vi "GraphCom.vi"() -> ()   [LabVIEW 2019]
uses:
  MessageFormat1.ctl
  <vilib>/Instr/_visa.llb/VISA Configure Serial Port (Instr).vi
panel:
  in  "Tab Control":enum32{"Alcohol Test", "Configuration"}(tab)
  out "Horizontal Graduated Bar":u8(slide) scale=0.0..100.0
  out "RxData As Number":u32
  in  "Start Test":bool
  in  "stop":bool
  out "RxData Log":string
  in  "Disconnect from Arduino":bool
  in  "Connect to Arduino":bool
  in  "VISA resource name":refnum<visa-resource-name>
  out "Connected":bool
  out "Receiving Data":bool
  out "Input buffer":string
  in  "Stop Acquisition":bool
  # "Dades rebudes per UART"
  # "Dades transportades al Consumer Loop"
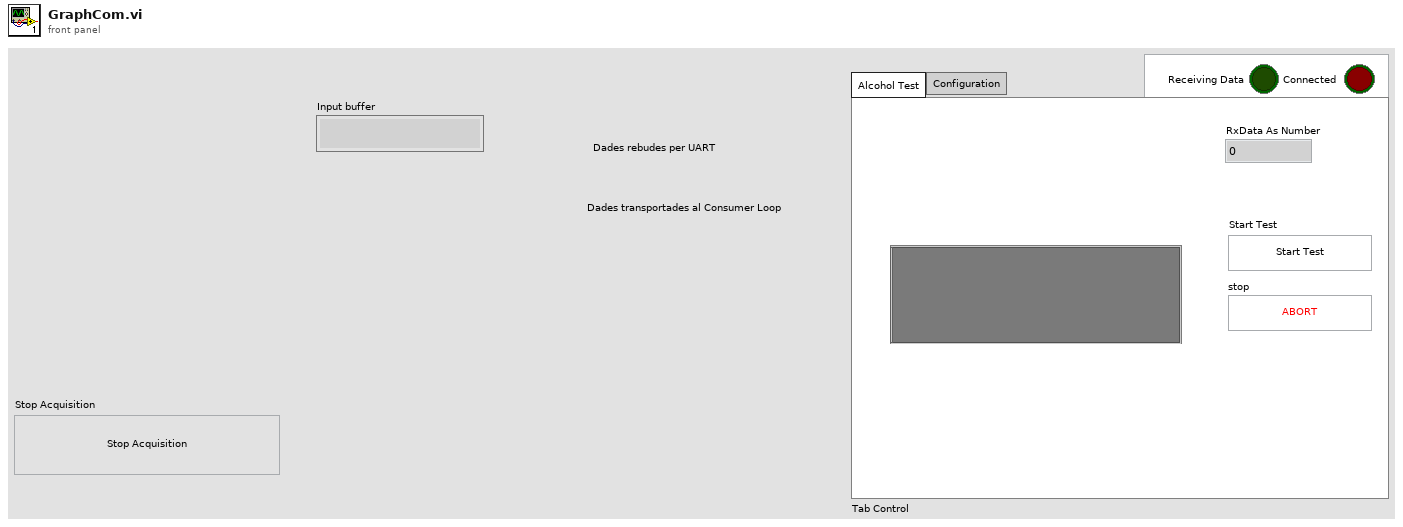
[diagram p1: front panel]
types:
  T1 = typedef "MessageFormat1.ctl" = cluster{"Consumer State":string, "RxData":string, "error constant":errorcluster, "Connected":bool, "Receiving Data":bool, "Producer State ":string}
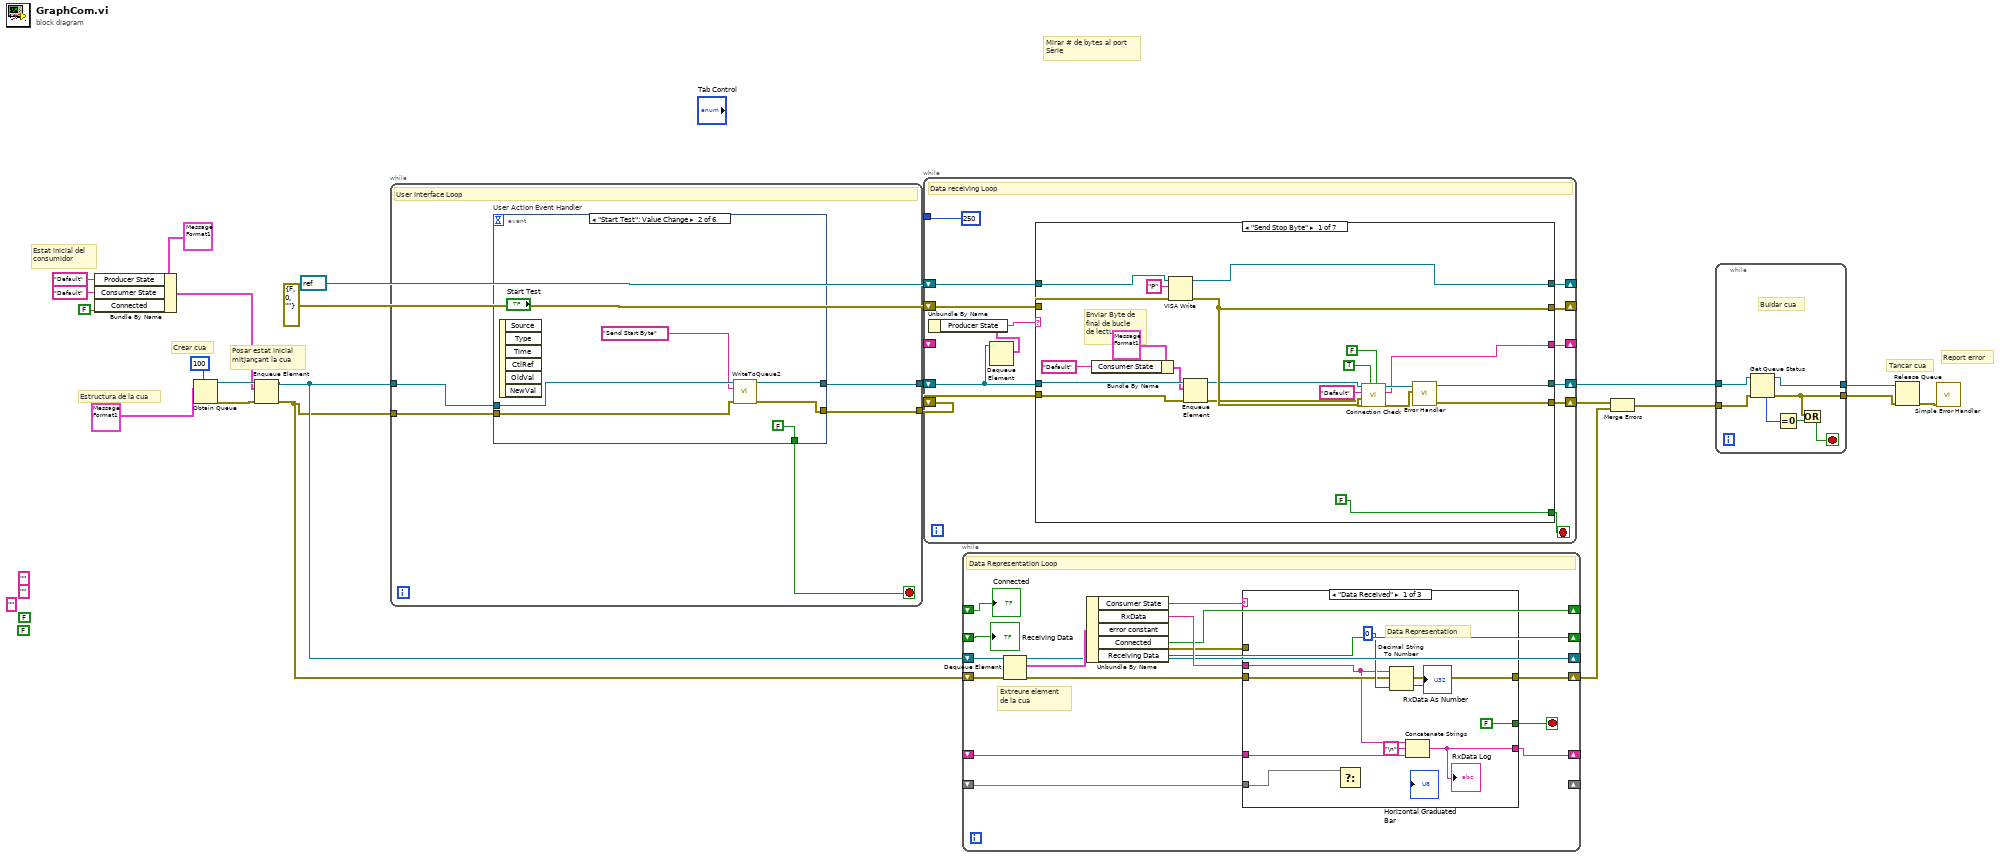
[diagram p0: block diagram]
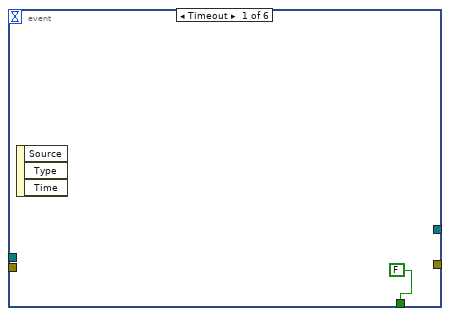
[diagram p2: hidden frame]
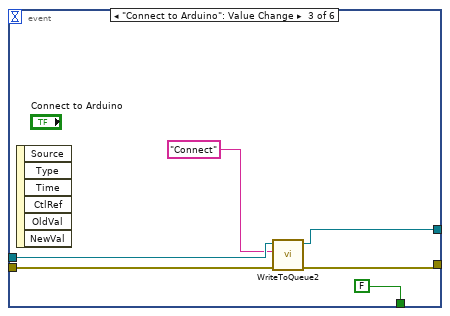
[diagram p3: hidden frame]
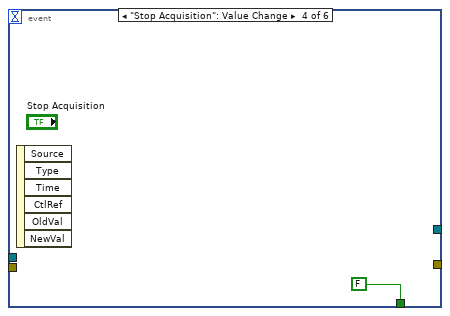
[diagram p4: hidden frame]
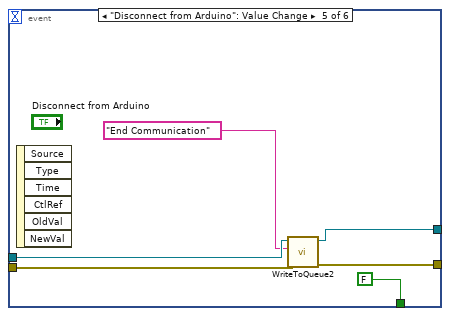
[diagram p5: hidden frame]
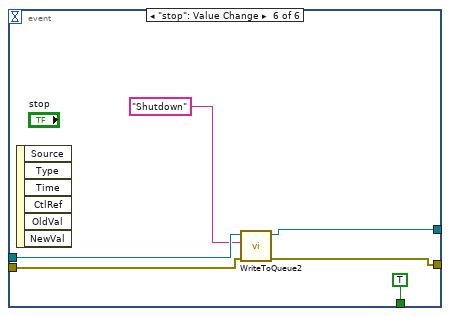
[diagram p6: hidden frame]
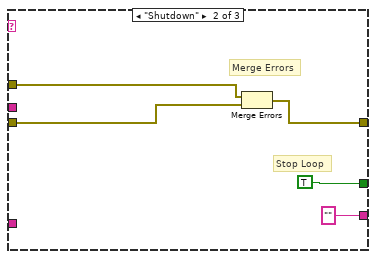
[diagram p7: hidden frame]
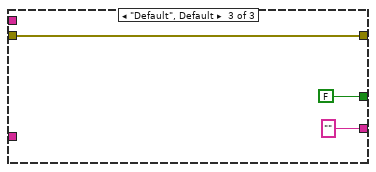
[diagram p8: hidden frame]
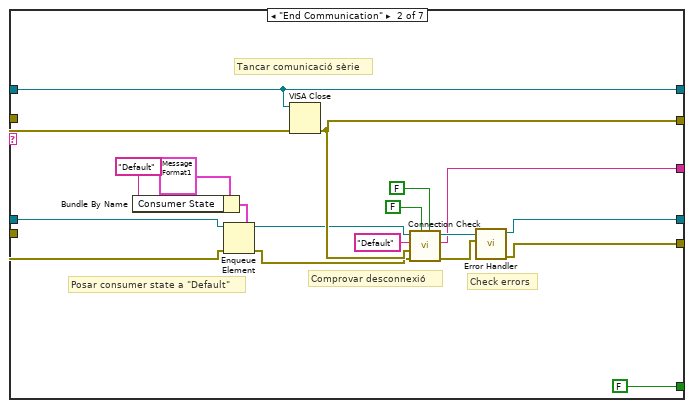
[diagram p9: hidden frame]
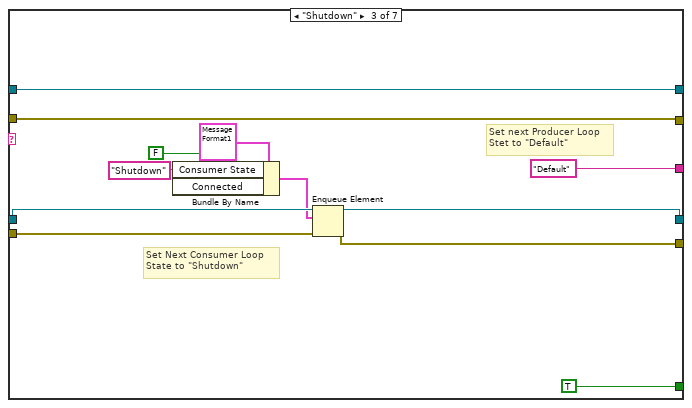
[diagram p10: hidden frame]
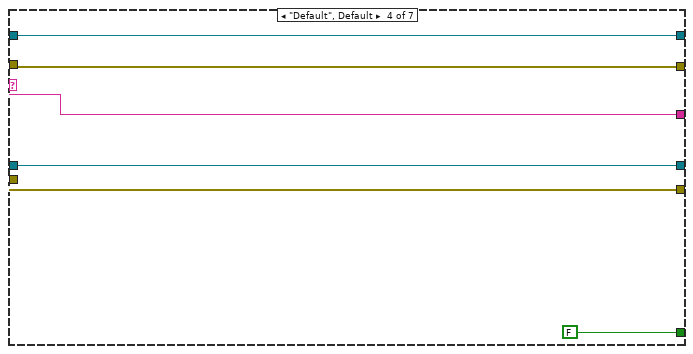
[diagram p11: hidden frame]
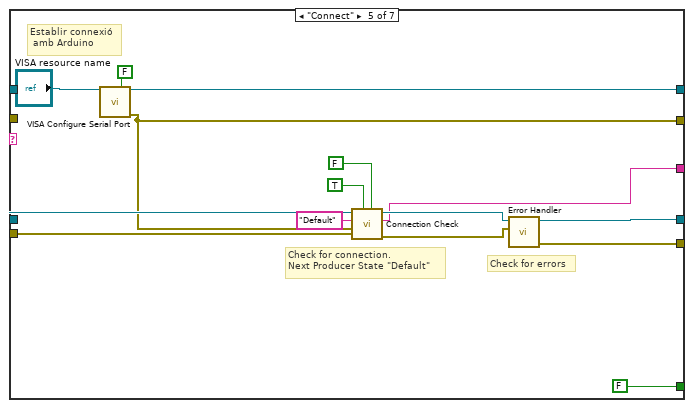
[diagram p12: hidden frame]
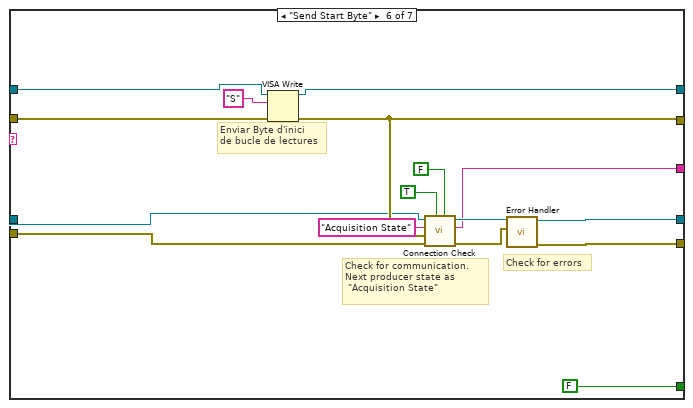
[diagram p13: hidden frame]
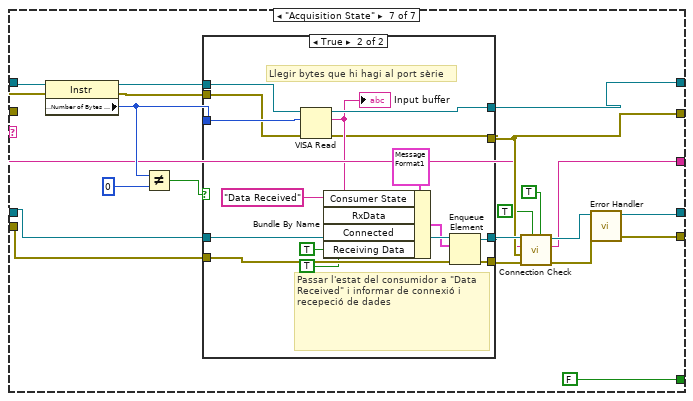
[diagram p14: hidden frame]
diagram:
  (unwired) "" ("Producer State")
  (unwired) FALSE ("Receiving Data")
  (unwired) FALSE ("Connected")
  (unwired) "" ("Consumer State")
  (unwired) "" ("Producer State")
  # "Tancar cua"
  # "Report error"
  # "Posar estat inicial \nmitjançant la cua"
  # "Crear cua"
  # "Mirar # de bytes al port\nSèrie"
  # "Estat inicial del \nconsumidor"
  # "Estructura de la cua"
  n1 = Bundle By Name(cluster=T1 {"Consumer State"="Consumer State", "RxData"="Received Data", "error constant"={"status"=FALSE, "code"=0, "source"=""}, "Connected"=FALSE, "Receiving Data"=FALSE, "Producer State "="Producer State"} ("Queue Definition"), "Producer State"="Default", "Consumer State"="Default", "Connected"=FALSE) -> (w15:T1)
  n2 = Obtain Queue(max queue size (-1, unlimited)=100, element data type=T1 {"Consumer State"="Consumer State", "RxData"="Received Data", "error constant"={"status"=FALSE, "code"=0, "source"=""}, "Connected"=FALSE, "Receiving Data"=FALSE, "Producer State "="Producer State"} ("Queue Definition")) -> (queue out=w17:refnum<queue>, error out=w18:errorcluster)  [unwired: 3 in, 1 out]
  n3 = Enqueue Element(queue=w17, element=w15, error in (no error)=w18) -> (queue out=w4:refnum<queue>, error out=w3:errorcluster)  [unwired: 1 in, 1 out]
  n4 = while {
    tunnel: w4 -> [w27]
    tunnel: w3 -> [w26]
    tunnel: [w25] -> w2
    tunnel: [w24] -> w1
    stop <- w23 stop-if-true
    # "User Interface Loop"
    n5 = event "User Action Event Handler" shown="[1] \"Start Test\": Value Change" {
      selector: _ -> [_ _ _ _ _ _]
      dyn-events: _ -> [_ _ _ _ _ _]
      timeout: _ -> [_ _ _ _ _ _]
      tunnel: w27 -> [_ w33 w40 _ w47 w52]
      tunnel: w26 -> [_ w34 w39 _ w46 w53]
      tunnel: [_ w32 w37 _ w44 w51] -> w25
      tunnel: [_ w31 w38 _ w43 w50] -> w24
      tunnel: [FALSE FALSE FALSE FALSE FALSE TRUE] -> w23
      event Timeout {
        n6 = event-data() -> ()  [unwired: 1 in, 3 out]
      }
      event "Start Test": Value Change {
        n7 = event-data() -> ()  [unwired: 1 in, 6 out]
        n8 = call "WriteToQueue2.vi"("error in (no error)"=w34, "Producer State"="Send Start Byte", "queue"=w33) -> ("error out"=w31:errorcluster, "queue out"=w32:refnum<queue>)  [unwired: 7 in]
      }
      event "Connect to Arduino": Value Change {
        n9 = event-data() -> ()  [unwired: 1 in, 6 out]
        n10 = call "WriteToQueue2.vi"("error in (no error)"=w39, "Producer State"="Connect" ("f"), "queue"=w40) -> ("error out"=w38:errorcluster, "queue out"=w37:refnum<queue>)  [unwired: 7 in]
      }
      event "Stop Acquisition": Value Change {
        n11 = event-data() -> ()  [unwired: 1 in, 6 out]
      }
      event "Disconnect from Arduino": Value Change {
        n12 = event-data() -> ()  [unwired: 1 in, 6 out]
        n13 = call "WriteToQueue2.vi"("error in (no error)"=w46, "Producer State"="End Communication" ("Producer State Out"), "queue"=w47) -> ("error out"=w43:errorcluster, "queue out"=w44:refnum<queue>)  [unwired: 7 in]
      }
      event "stop": Value Change {
        n14 = event-data() -> ()  [unwired: 1 in, 6 out]
        n15 = call "WriteToQueue2.vi"("error in (no error)"=w53, "Producer State"="Shutdown", "queue"=w52) -> ("error out"=w50:errorcluster, "queue out"=w51:refnum<queue>)  [unwired: 7 in]
      }
    }
  }
  n16 = while {
    shift-right: [w66] -> _
    shift-left: refnum<visa-resource-name> refnum ("VISA resource name out") -> [w63]
    shift-right: [w65] -> _
    shift-left: errorcluster {"status"=FALSE, "code"=0, "source"=""} ("error out") -> [w62]
    shift-right: [w58] -> w10
    shift-left: w2 -> [w56]
    shift-right: [w59] -> w21
    shift-left: w1 -> [w61]
    shift-right: [w64] -> _
    shift-left: _ -> [_]
    tunnel: [250] -> _
    stop <- w60 stop-if-true
    # "Data receiving Loop"
    n17 = Dequeue Element(queue=w56) -> (element=w55:T1)  [unwired: 2 in, 3 out]
    n18 = Unbundle By Name(w55) -> ("Producer State"=w54:string)
    n19 = case shown="\"Send Stop Byte\"" w54 {
      selector: w54 -> [_ _ _ w121 _ _ w159]
      tunnel: [w83 w104 w117 w122 w136 w152 w172] -> w66
      tunnel: [w74 w97 w116 w123 w130 w146 w162] -> w65
      tunnel: [w79 w96 w111 w124 w131 w150 w161] -> w59
      tunnel: [w80 w95 w112 w119 w132 w149 w160] -> w58
      tunnel: [FALSE FALSE TRUE FALSE FALSE FALSE FALSE] -> w60
      tunnel: [w78 w98 "Default" ("f") w121 w128 w145 w158] -> w64
      tunnel: w63 -> [w84 w104 w117 w122 _ w153 w177]
      tunnel: w62 -> [w85 w105 w116 w123 _ w154 w176]
      tunnel: w61 -> [w72 w92 w110 w124 w135 w143 w170]
      tunnel: w56 -> [w71 w93 w114 w119 w134 w142 w171]
      frame "Send Stop Byte" {
        # "Enviar Byte de \nfinal de bucle \nde lectures"
        n20 = Bundle By Name(cluster=T1 {"Consumer State"="Consumer State", "RxData"="Received Data", "error constant"={"status"=FALSE, "code"=0, "source"=""}, "Connected"=FALSE, "Receiving Data"=FALSE, "Producer State "="Consumer State"} ("Queue Definition"), "Consumer State"="Default") -> (w69:T1)
        n21 = VISA Write(VISA resource name=w84, write buffer="P", error in (no error)=w85) -> (VISA resource name out=w83:refnum<visa-resource-name>, error out=w74:errorcluster)  [unwired: 1 out]
        n22 = Enqueue Element(queue=w71, element=w69, error in (no error)=w72) -> (queue out=w70:refnum<queue>, error out=w73:errorcluster)  [unwired: 1 in, 1 out]
        n23 = call "Connection Check.vi"("Queue in"=w70, "Producer State In"="Default", "error in"=w74, "error in (no error)"=w73, "Connected"=TRUE, "Receiving Data"=FALSE) -> ("Queue out"=w82:refnum<queue>, "Producer State Out"=w78:string, "error out"=w81:errorcluster)  [unwired: 2 in]
        n24 = call "Error Handler.vi"("error in"=w81, "Queue in"=w82) -> ("error out"=w79:errorcluster, "Queue out"=w80:refnum<queue>)  [unwired: 8 in]
      }
      frame "End Communication" {
        # "Tancar comunicació sèrie"
        # "Check errors"
        # "Comprovar desconnexió"
        # "Posar consumer state a \"Default\""
        n25 = Bundle By Name(cluster=T1 {"Consumer State"="Consumer State", "RxData"="Received Data", "error constant"={"status"=FALSE, "code"=0, "source"=""}, "Connected"=FALSE, "Receiving Data"=FALSE, "Producer State "="Consumer State"} ("Queue Definition"), "Consumer State"="Default") -> (w88:T1)
        n26 = Enqueue Element(queue=w93, element=w88, error in (no error)=w92) -> (queue out=w94:refnum<queue>, error out=w91:errorcluster)  [unwired: 1 in, 1 out]
        n27 = VISA Close(VISA resource name=w104, error in (no error)=w105) -> (error out=w97:errorcluster)
        n28 = call "Connection Check.vi"("Queue in"=w94, "Producer State In"="Default", "error in"=w97, "error in (no error)"=w91, "Connected"=FALSE, "Receiving Data"=FALSE) -> ("Queue out"=w103:refnum<queue>, "Producer State Out"=w98:string, "error out"=w102:errorcluster)  [unwired: 2 in]
        n29 = call "Error Handler.vi"("error in"=w102, "Queue in"=w103) -> ("error out"=w96:errorcluster, "Queue out"=w95:refnum<queue>)  [unwired: 8 in]
      }
      frame "Shutdown" {
        # "Set next Producer Loop\nStet to \"Default\""
        # "Set Next Consumer Loop\nState to \"Shutdown\""
        n30 = Bundle By Name(cluster=T1 {"Consumer State"="Consumer State", "RxData"="Received Data", "error constant"={"status"=FALSE, "code"=0, "source"=""}, "Connected"=FALSE, "Receiving Data"=FALSE, "Producer State "="Consumer State"} ("Queue Definition"), "Consumer State"="Shutdown", "Connected"=FALSE) -> (w108:T1)
        n31 = Enqueue Element(queue=w114, element=w108, error in (no error)=w110) -> (queue out=w112:refnum<queue>, error out=w111:errorcluster)  [unwired: 1 in, 1 out]
      }
      frame "Default", Default {
      }
      frame "Connect" {
        # "Check for errors"
        # "Check for connection.\nNext Producer State \"Default\""
        # "Establir connexió\n amb Arduino"
        n32 = call-poly "VISA Configure Serial Port"("VISA resource name"="VISA resource name", "Enable Termination\nChar (T)"=FALSE ("Enable Termination\nChar (T)")) -> ("VISA resource name out"=w136:refnum<visa-resource-name>, "error out"=w130:errorcluster)  [unwired: 12 in]
        n33 = call "Connection Check.vi"("Queue in"=w134, "Producer State In"="Default", "error in"=w130, "error in (no error)"=w135, "Connected"=TRUE, "Receiving Data"=FALSE) -> ("Queue out"=w133:refnum<queue>, "Producer State Out"=w128:string, "error out"=w129:errorcluster)  [unwired: 2 in]
        n34 = call "Error Handler.vi"("error in"=w129, "Queue in"=w133) -> ("error out"=w131:errorcluster, "Queue out"=w132:refnum<queue>)  [unwired: 8 in]
      }
      frame "Send Start Byte" {
        # "Check for errors"
        # "Check for communication.\nNext producer state as\n \"Acquisition State\""
        # "Enviar Byte d'inici\nde bucle de lectures"
        n35 = VISA Write(VISA resource name=w153, write buffer="S", error in (no error)=w154) -> (VISA resource name out=w152:refnum<visa-resource-name>, error out=w146:errorcluster)  [unwired: 1 out]
        n36 = call "Connection Check.vi"("Queue in"=w142, "Producer State In"="Acquisition State", "error in"=w146, "error in (no error)"=w143, "Connected"=TRUE, "Receiving Data"=FALSE) -> ("Queue out"=w147:refnum<queue>, "Producer State Out"=w145:string, "error out"=w148:errorcluster)  [unwired: 2 in]
        n37 = call "Error Handler.vi"("error in"=w148, "Queue in"=w147) -> ("error out"=w150:errorcluster, "Queue out"=w149:refnum<queue>)  [unwired: 8 in]
      }
      frame "Acquisition State" {
        n38 = property class="Instr"(reference=w177, error in=w176) -> (reference out=w169:refnum<visa-resource-name>, error out=w168:errorcluster, "Serial Settings:Number of Bytes at Serial Port"=w175:u32)
        n39 = Not Equal?(x=w175, y=u32 0) -> (x != y?=w173:bool)
        n40 = case shown="True" w173 {
          tunnel: [w180 w196] -> w172
          tunnel: [w179 w186] -> w162
          tunnel: [w181 w185] -> w164
          tunnel: w175 -> [_ w193]
          tunnel: w171 -> [w181 w189]
          tunnel: w170 -> [w178 w190]
          tunnel: w169 -> [w180 w192]
          tunnel: w168 -> [w179 w191]
          tunnel: [w178 w184] -> w163
          frame False {
          }
          frame True {
            # "Passar l'estat del consumidor a \"Data Received\" i informar de connexió i recepeció de dades"
            # "Llegir bytes que hi hagi al port sèrie"
            n41 = VISA Read(VISA resource name=w192, byte count=w193, error in (no error)=w191) -> (VISA resource name out=w196:refnum<visa-resource-name>, read buffer=w195:string, error out=w186:errorcluster)  [unwired: 1 out]
            "Input buffer" <- w195
            n42 = Bundle By Name(cluster=T1 {"Consumer State"="Consumer State", "RxData"="Received Data", "error constant"={"status"=FALSE, "code"=0, "source"=""}, "Connected"=FALSE, "Receiving Data"=FALSE, "Producer State "="Consumer State"} ("Queue Definition"), "Consumer State"="Data Received" ("Next State"), "RxData"=w195, "Connected"=TRUE, "Receiving Data"=TRUE) -> (w187:T1)
            n43 = Enqueue Element(queue=w189, element=w187, error in (no error)=w190) -> (queue out=w185:refnum<queue>, error out=w184:errorcluster)  [unwired: 1 in, 1 out]
          }
        }
        n44 = call "Connection Check.vi"("Queue in"=w164, "Producer State In"=w159, "error in"=w162, "error in (no error)"=w163, "Connected"=TRUE, "Receiving Data"=TRUE) -> ("Queue out"=w166:refnum<queue>, "Producer State Out"=w158:string, "error out"=w165:errorcluster)  [unwired: 2 in]
        n45 = call "Error Handler.vi"("error in"=w165, "Queue in"=w166) -> ("error out"=w161:errorcluster, "Queue out"=w160:refnum<queue>)  [unwired: 8 in]
      }
    }
  }
  n46 = while {
    shift-right: [w201] -> w19
    shift-left: w3 -> [w212]
    shift-right: [w208] -> _
    shift-left: w4 -> [w213]
    shift-right: [w205] -> _
    shift-left: _ -> [w204]
    shift-right: [w203] -> _
    shift-left: _ -> [w202]
    shift-right: [w198] -> _
    shift-left: _ -> [w199]
    shift-right: _ -> [_]
    shift-left: _ -> [w197]
    stop <- w207 stop-if-true
    # "Extreure element \nde la cua"
    # "Data Representation Loop"
    n47 = Dequeue Element(queue=w213, error in (no error)=w212) -> (queue out=w208:refnum<queue>, element=w211:T1, error out=w200:errorcluster)  [unwired: 1 in, 1 out]
    n48 = Unbundle By Name(w211) -> ("Consumer State"=w209:string, "RxData"=w210:string, "error constant"=w206:errorcluster, "Connected"=w205:bool, "Receiving Data"=w203:bool)
    n49 = case shown="\"Data Received\"" w209 {
      tunnel: w210 -> [w217 _ _]
      tunnel: [FALSE TRUE FALSE] -> w207
      tunnel: w206 -> [_ w226 _]
      tunnel: [w220 w227 w230] -> w201
      tunnel: w200 -> [w220 w225 w230]
      tunnel: w199 -> [w219 _ _]
      tunnel: [w218 "" ""] -> w198
      tunnel: w197 -> [w214 _ _]
      frame "Data Received" {
        # "Data Representation"
        n50 = Select(t=w214) -> (f=w215:dbl)  [unwired: 1 in, 1 out]
        n51 = Decimal String To Number(string=w217, default (0L)=u32 0) -> (number=→"RxData As Number":u32)  [unwired: 1 in, 1 out]
        n52 = Concatenate Strings(w217, "\n" ("string"), w219) -> (w218:string)
        "RxData Log" <- w218
      }
      frame "Shutdown" {
        # "Stop Loop"
        # "Merge Errors"
        n53 = Merge Errors(w226, w225) -> (w227:errorcluster)
      }
      frame "Default", Default {
      }
    }
    "Receiving Data" <- w202
    "Connected" <- w204
  }
  n54 = Merge Errors(w21, w19) -> (w9:errorcluster)
  n55 = while {
    tunnel: w10 -> [w238]
    tunnel: w9 -> [w237]
    tunnel: [w233] -> w8
    tunnel: [w236] -> w7
    stop <- w232 stop-if-true
    # "Buidar cua"
    n56 = Get Queue Status(queue=w238, error in (no error)=w237) -> (queue out=w236:refnum<queue>, error out=w233:errorcluster, # elements in queue=w235:i32)  [unwired: 1 in, 5 out]
    n57 = Equal To 0?(x=w235) -> (x = 0?=w234:bool)
    n58 = Or(x=w233, y=w234) -> (x .or. y?=w232:bool)
  }
  n59 = Release Queue(queue=w7, error in (no error)=w8) -> (error out=w6:errorcluster)  [unwired: 1 in, 2 out]
  n60 = call <vilib>:"Simple Error Handler.vi"("error in (no error)"=w6) -> ()  [unwired: 4 in, 5 out]
